vi "消除电流零偏.vi"   [LabVIEW 2020]
uses:
  <vilib>/Analysis/baseanly.llb/Mean (DBL).vi
  <vilib>/Utility/file.llb/Read Delimited Spreadsheet (DBL).vi
  <vilib>/Utility/file.llb/Write Delimited Spreadsheet (DBL).vi
  <vilib>/Analysis/NI_AALBase.lvlib
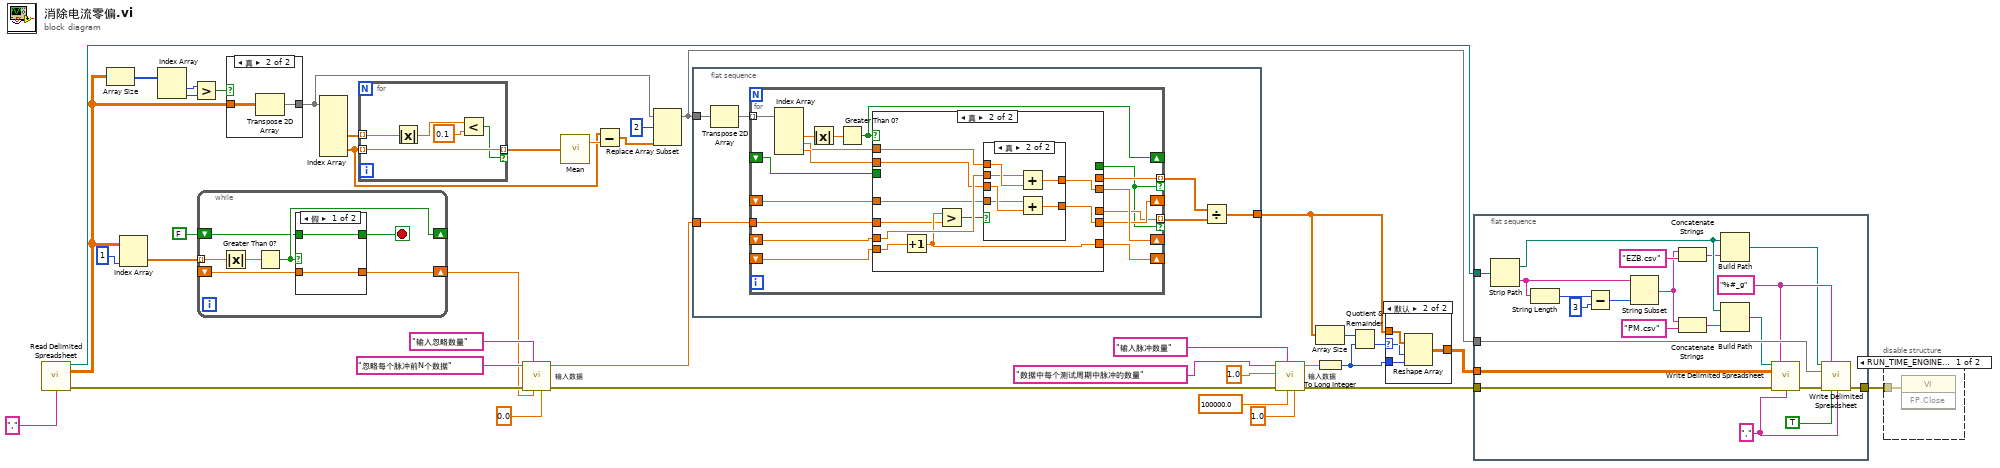
[diagram p0: block diagram]
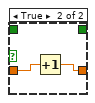
[diagram p2: hidden frame]
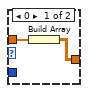
[diagram p4: hidden frame]
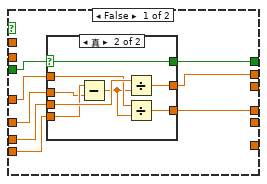
[diagram p5: hidden frame]
diagram:
  n1 = call-poly <vilib>:"Read Delimited Spreadsheet.vi"("delimiter (\\t)"="," ("delimiter (\\t)")) -> ("new file path (Not A Path if cancelled)"=w25:path, "all rows"=w23:dbl[][], "error out"=w22:errorcluster)  [unwired: 9 in, 3 out]
  n2 = Array Size(array=w23) -> (size(s)=w29:i32[])
  n3 = Index Array(array=w23, index (col)=1 ("禁用的索引 (列)")) -> (element=w4:dbl[])  [unwired: 1 in]
  n4 = Index Array(array=w29) -> (element #1=w28:i32, element #2=w27:i32)  [unwired: 2 in]
  n5 = Greater?(x=w28, y=w27) -> (0:w26:bool)
  n6 = while {
    shift-right: [w44] -> w6
    shift-left: _ -> [w45]
    shift-right: [w43] -> _
    shift-left: FALSE -> [w42]
    tunnel: w4 -> [w39] mode=indexing
    stop <- w40 stop-if-true
    n7 = Absolute Value(x=w39) -> (abs(x)=w41:dbl)
    n8 = Greater Than 0?(x=w41) -> (x > 0?=w43:bool)
    n9 = case shown="假" w43 {
      tunnel: w45 -> [w46 w49]
      tunnel: [w46 w48] -> w44
      tunnel: w42 -> [w47 _]
      tunnel: [w47 _] -> w40
      frame False {
      }
      frame True {
        n10 = Increment(x=w49) -> (x+1=w48:dbl)
      }
    }
  }
  n11 = case shown="真" w26 {
    tunnel: [w50 w52] -> w30
    tunnel: w23 -> [w50 w51]
    frame False {
    }
    frame True {
      n12 = Transpose 2D Array(2D array=w51) -> (transposed array=w52:dbl[][])
    }
  }
  n13 = Index Array(array=w30) -> (element #2=w32:dbl[], element #3=w35:dbl[])  [unwired: 6 in, 1 out]
  n14 = for {
    tunnel: w32 -> [w57] mode=indexing
    tunnel: w35 -> [w55] mode=indexing
    tunnel: [w55] -> w37 mode=indexing if=w54
    n15 = Absolute Value(x=w57) -> (abs(x)=w53:dbl)
    n16 = Less?(x=w53, y=0.1) -> (x < y?=w54:bool)
  }
  n17 = call "输入数据.vi"("数据输入界限:最小值"=0.0, "数据输入界限:最大值"=w6, "前面板窗口:标题"="输入忽略数量", "错误输入（无错误）"=w22, "提示"="忽略每个脉冲前N个数据") -> ("错误输出"=w20:errorcluster, "输入数据"=w21:dbl)  [unwired: 5 in]
  n18 = call-poly <vilib>:"Mean.vi"("X"=w37) -> ("mean"=w36:dbl)  [unwired: 1 out]
  n19 = Subtract(x=w35, y=w36) -> (x-y=w33:dbl[])
  n20 = Replace Array Subset(array=w30, new element=w33, index (row)=2 ("索引 (行)")) -> (w24:dbl[][])  [unwired: 1 in]
  n21 = flat-sequence {
    tunnel: [w61] -> w14
    tunnel: w24 -> [w60]
    tunnel: w21 -> [w58]
    frame #0 {
      n22 = Transpose 2D Array(2D array=w60) -> (transposed array=w59:dbl[][])
      n23 = for {
        shift-right: [w80] -> _
        shift-left: _ -> [w79]
        shift-right: [w78] -> _
        shift-left: _ -> [w77]
        shift-right: [w75] -> _
        shift-left: _ -> [w76]
        shift-right: [w74] -> _
        shift-left: _ -> [w73]
        tunnel: [w72] -> w63 mode=indexing if=w69
        tunnel: [w71] -> w62 mode=indexing if=w69
        tunnel: w58 -> [w68]
        tunnel: w59 -> [w67] mode=indexing
        n24 = Index Array(array=w67) -> (element #2=w64:dbl, element #3=w65:dbl, element #4=w66:dbl)  [unwired: 4 in, 1 out]
        n25 = Absolute Value(x=w64) -> (abs(x)=w70:dbl)
        n26 = Greater Than 0?(x=w70) -> (x > 0?=w74:bool)
        n27 = case shown="真" w74 {
          tunnel: w65 -> [_ w106]
          tunnel: w66 -> [_ w103]
          tunnel: [_ w105] -> w80
          tunnel: w79 -> [w87 w104]
          tunnel: [_ w102] -> w78
          tunnel: w77 -> [w83 w101]
          tunnel: w76 -> [w86 w100]
          tunnel: [_ w99] -> w75
          tunnel: w73 -> [w88 _]
          tunnel: [w85 _] -> w72
          tunnel: [w84 _] -> w69
          tunnel: [w82 _] -> w71
          tunnel: w68 -> [w81 w98]
          frame False {
            n28 = case shown="真" w88 {
              selector: w88 -> [_ w94]
              tunnel: w87 -> [_ w96]
              tunnel: w86 -> [_ w90]
              tunnel: [_ w95] -> w85
              tunnel: [_ w94] -> w84
              tunnel: w83 -> [_ w93]
              tunnel: [_ w92] -> w82
              tunnel: w81 -> [_ w89]
              frame False {
              }
              frame True {
                n29 = Subtract(x=w90, y=w89) -> (x-y=w91:dbl)
                n30 = Divide(x=w96, y=w91) -> (x/y=w95:dbl)
                n31 = Divide(x=w93, y=w91) -> (x/y=w92:dbl)
              }
            }
          }
          frame True {
            n32 = Increment(x=w100) -> (x+1=w99:dbl)
            n33 = Greater?(x=w99, y=w98) -> (0:w97:bool)
            n34 = case shown="真" w97 {
              tunnel: w106 -> [_ w112]
              tunnel: [_ w111] -> w105
              tunnel: w104 -> [_ w110]
              tunnel: w103 -> [_ w109]
              tunnel: [_ w108] -> w102
              tunnel: w101 -> [_ w107]
              frame False {
              }
              frame True {
                n35 = Add(x=w110, y=w112) -> (x+y=w111:dbl)
                n36 = Add(x=w107, y=w109) -> (x+y=w108:dbl)
              }
            }
          }
        }
      }
      n37 = Divide(x=w63, y=w62) -> (x/y=w61:dbl[])
    }
  }
  n38 = call "输入数据.vi"("数据输入界限:最小值"=1.0, "数据输入界限:最大值"=100000.0, "前面板窗口:标题"="输入脉冲数量", "错误输入（无错误）"=w20, "默认值"=1.0, "提示"="数据中每个测试周期中脉冲的数量") -> ("错误输出"=w19:errorcluster, "输入数据"=w11:dbl)  [unwired: 4 in]
  n39 = Array Size(array=w14) -> (size(s)=w13:i32)
  n40 = To Long Integer(number=w11) -> (32bit integer=w1:i32)
  n41 = Quotient & Remainder(x=w13, y=w1) -> (floor(x/y)=w12:i32)  [unwired: 1 out]
  n42 = case shown="默认" w12 {
    selector: w12 -> [_ w117]
    tunnel: w14 -> [w114 w118]
    tunnel: w1 -> [_ w116]
    tunnel: [w113 w115] -> w10
    frame 0 {
      n43 = Build Array(w114) -> (w113:dbl[][])
    }
    frame Default {
      n44 = Reshape Array(w118, w117, w116) -> (w115:dbl[][])
    }
  }
  n45 = flat-sequence {
    tunnel: w24 -> [w139]
    tunnel: w19 -> [w136]
    tunnel: [w133] -> w31
    tunnel: w25 -> [w132]
    tunnel: w10 -> [w119]
    frame #0 {
      w138 = "," ("delimiter (\\t)")
      w137 = "%#_g" ("format (%.3f)")
      n46 = Strip Path(path=w132) -> (stripped path=w129:path, name=w123:string)
      n47 = String Length(string=w123) -> (length=w122:i32)
      n48 = Subtract(x=w122, y=3) -> (x-y=w120:i32)
      n49 = String Subset(string=w123, length (rest)=w120) -> (substring=w124:string)  [unwired: 1 in]
      n50 = Concatenate Strings(w124, "EZB.csv" ("字符串")) -> (w128:string)
      n51 = Concatenate Strings(w124, "PM.csv" ("字符串")) -> (w127:string)
      n52 = Build Path(base path=w129, name or relative path=w128) -> (appended path=w131:path)
      n53 = Build Path(base path=w129, name or relative path=w127) -> (appended path=w130:path)
      n54 = call-poly <vilib>:"Write Delimited Spreadsheet.vi"("file path (dialog if empty)"=w130, "format (%.3f)"=w137, "2D data"=w119, "error in (no error)"=w136, "delimiter (\\t)"=w138) -> ("error out"=w135:errorcluster)  [unwired: 9 in, 1 out]
      n55 = call-poly <vilib>:"Write Delimited Spreadsheet.vi"("file path (dialog if empty)"=w131, "format (%.3f)"=w137, "2D data"=w139, "error in (no error)"=w135, "transpose? (no:F)"=TRUE, "delimiter (\\t)"=w138) -> ("error out"=w133:errorcluster)  [unwired: 8 in, 1 out]
    }
  }
  n56 = disable-structure shown="RUN_TIME_ENGINE==True" {
    disable-tunnel: w31 -> [w140 _]
    frame condition #0 {
      n57 = invoke class="VI" method="FP.Close"(error in=w140) -> ()  [unwired: 2 in, 3 out]
    }
    frame condition #1 (active) {
    }
  }
